vi "Get Class Indent Order.vi"(11 "Tree Sorted Array":T1(array[cluster])) -> (2 "Indent":u32[](array[numeric]), 3 "Tree Sorted Array Out":T1(array[cluster]))   [LabVIEW 2023]
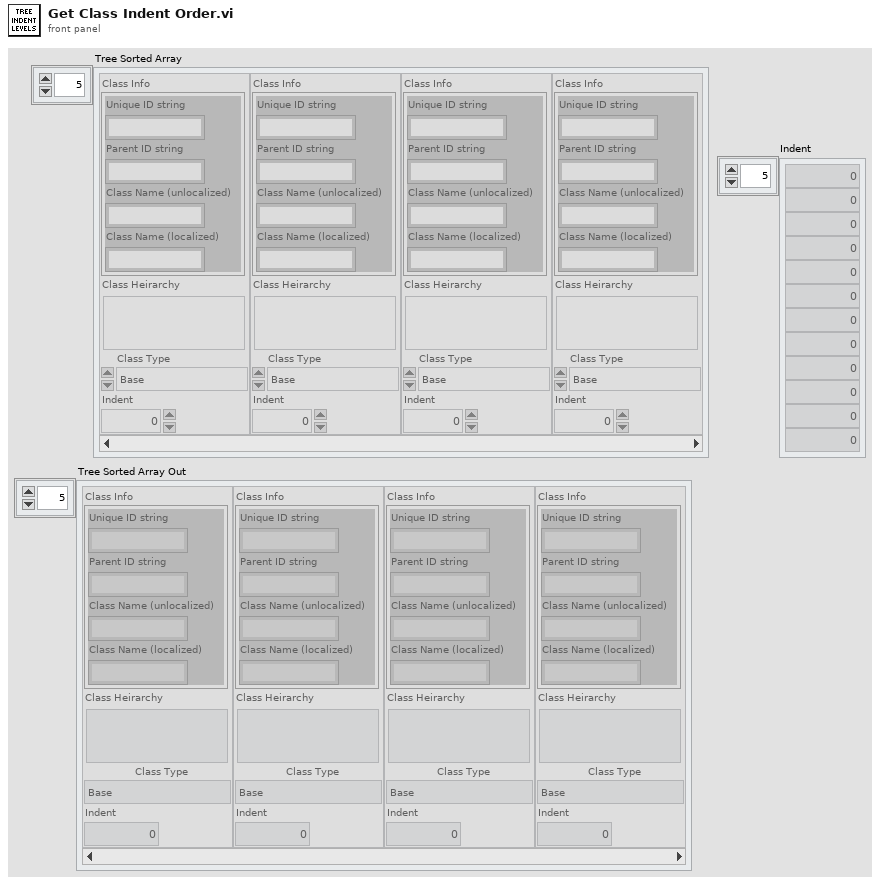
[diagram p1: front panel]
types:
  T1 = cluster{"Class Info":cluster{"Unique ID string":string, "Parent ID string":string, "Class Name (unlocalized)":string, "Class Name (localized)":string}, "Class Heirarchy":string, "Class Type":enum16{"Unknown", "Base", "Scripting", "Private", "Deprecated", "None", "Divider"}, "Indent":u32}[]
  T2 = cluster{"Class Info":cluster{"Unique ID string":string, "Parent ID string":string, "Class Name (unlocalized)":string, "Class Name (localized)":string}, "Class Heirarchy":string, "Class Type":enum16{"Unknown", "Base", "Scripting", "Private", "Deprecated", "None", "Divider"}, "Indent":u32}
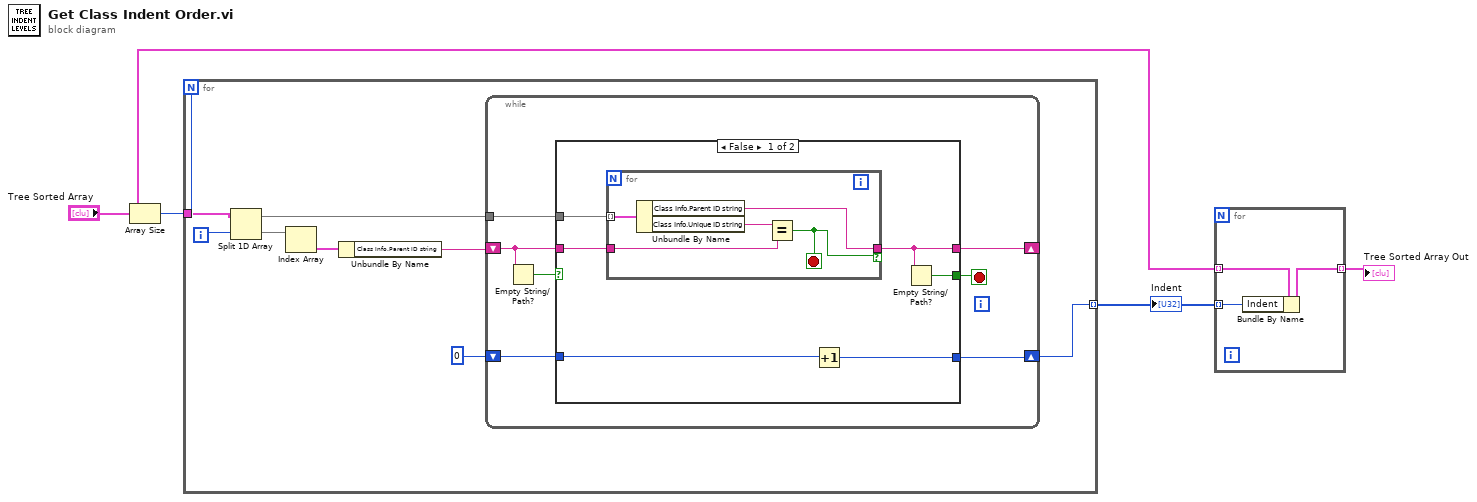
[diagram p0: block diagram]
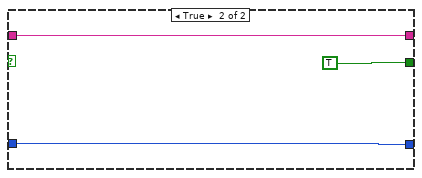
[diagram p2: hidden frame]
diagram:
  n1 = Array Size(array="Tree Sorted Array") -> (size(s)=w4:i32)
  n2 = for {
    N: w4 -> [_]
    tunnel: "Tree Sorted Array" -> [w12]
    tunnel: [w5] -> w2 mode=indexing
    i -> [w11]
    n3 = Split 1D Array(array=w12, index=w11) -> (first subarray=w10:T1, second subarray=w9:T1)
    n4 = Index Array(array=w9) -> (element=w8:T2)  [unwired: 1 in]
    n5 = Unbundle By Name(w8) -> ("Class Info.Parent ID string"=w7:string)
    n6 = while {
      tunnel: w10 -> [w19]
      shift-right: [w18] -> _
      shift-left: w7 -> [w16]
      shift-right: [w14] -> w5
      shift-left: 0 -> [w15]
      stop <- w17 stop-if-true
      n7 = Empty String/Path?(string/path=w16) -> (empty?=w13:bool)
      n8 = case shown="False" w13 {
        tunnel: w19 -> [w25 _]
        tunnel: [w24 w31] -> w18
        tunnel: [w23 TRUE] -> w17
        tunnel: w16 -> [w22 w31]
        tunnel: w15 -> [w21 w33]
        tunnel: [w20 w33] -> w14
        frame False {
          n9 = for {
            tunnel: w25 -> [w30] mode=indexing
            tunnel: [w28] -> w24 if=w27
            tunnel: w22 -> [w26]
            stop <- w27 stop-if-true
            n10 = Unbundle By Name(w30) -> ("Class Info.Parent ID string"=w28:string, "Class Info.Unique ID string"=w29:string)
            n11 = Equal?(x=w29, y=w26) -> (x = y?=w27:bool)
          }
          n12 = Increment(x=w21) -> (x+1=w20:i32)
          n13 = Empty String/Path?(string/path=w24) -> (empty?=w23:bool)
        }
        frame True {
        }
      }
    }
  }
  "Indent" <- w2
  n14 = for {
    tunnel: "Tree Sorted Array" -> [w36] mode=indexing
    tunnel: w2 -> [w35] mode=indexing
    tunnel: [w34] -> w1 mode=indexing
    n15 = Bundle By Name(cluster=w36, "Indent"=w35) -> (w34:T2)
  }
  "Tree Sorted Array Out" <- w1
